vi "Get Process LLB Actions.vi"(8 "error in (no error)":errorcluster {"code" format="Error %.0f"}, 11 "VIDoc Printer In":refnum<class "VIDoc Printer.lvclass">) -> (0 "error out":errorcluster {"code" format="Error %.0f"}, 2 "Process LLB Actions":T1[](array[typedef]), 3 "VIDoc Printer Out":refnum<class "VIDoc Printer.lvclass">)   [LabVIEW 2023, in "VIDoc Printer.lvlib" / "VIDoc Printer.lvclass"]
uses:
  VIDoc Printer.lvclass
  VIDoc Printer.lvclass/VIDoc Printer.ctl
  Controls/Process LLB Enum.ctl
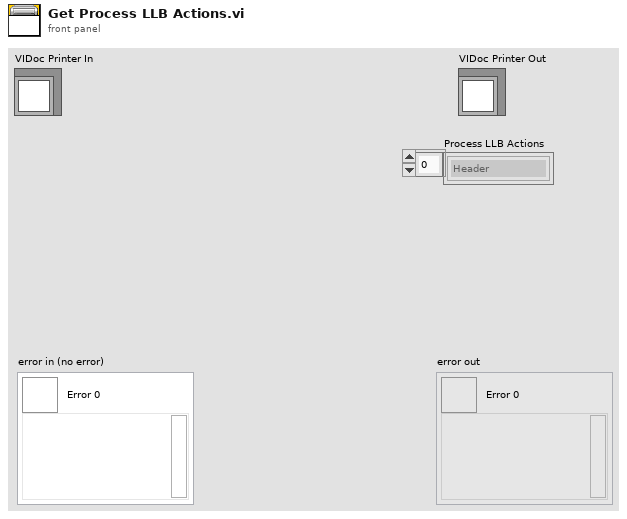
[diagram p1: front panel]
types:
  T1 = typedef "VIDoc Printer.lvlib/VIDoc Printer.lvclass/Process LLB Enum.ctl" = enum16{"Header", "By List", "Methods", "Controls"}
  T2 = typedef "VIDoc Printer.lvlib/Printer Settings.lvclass/Detail Level Enum.ctl" = enum16{"None", "Minimal", "Standard", "Full"}
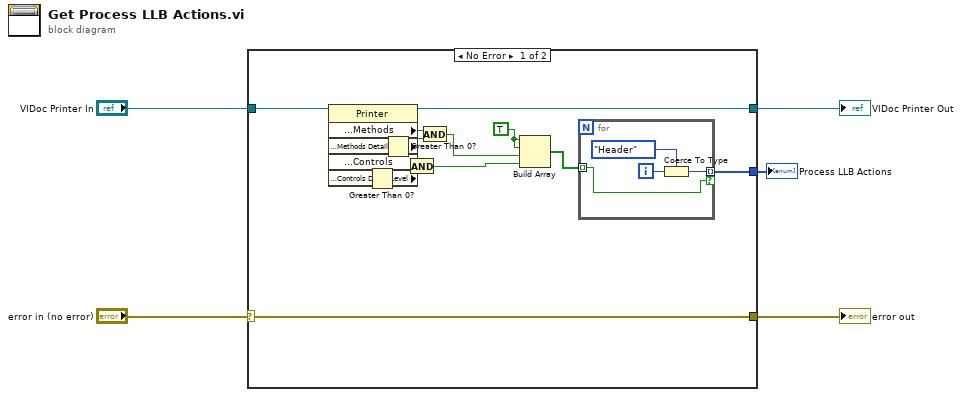
[diagram p0: block diagram]
diagram:
  n1 = case shown="No Error" "error in (no error)" {
    selector: "error in (no error)" -> [w19 w25]
    tunnel: [w19 w25] -> w4
    tunnel: [w16 w24] -> w2
    tunnel: "VIDoc Printer In" -> [w17 w24]
    tunnel: [w14 _] -> w1
    frame No Error {
      w6 = TRUE ("element")
      n2 = property class="Printer"(reference=w17) -> (reference out=w16:refnum<class "VIDoc Printer.lvclass">, "Properties:Settings:LLBs:Methods"=w18:bool, "Properties:Settings:LLBs:Methods Detail Level"=w13:T2, "Properties:Settings:LLBs:Controls"=w10:bool, "Properties:Settings:LLBs:Controls Detail Level"=w8:T2)  [unwired: 1 in, 1 out]
      n3 = Greater Than 0?(x=w8) -> (x > 0?=w9:bool)
      n4 = Greater Than 0?(x=w13) -> (x > 0?=w11:bool)
      n5 = And(x=w10, y=w9) -> (x .and. y?=w7:bool)
      n6 = And(x=w18, y=w11) -> (x .and. y?=w12:bool)
      n7 = Build Array(w6, w6, w12, w7) -> (w15:bool[])
      n8 = for {
        tunnel: w15 -> [w20] mode=indexing
        tunnel: [w21] -> w14 mode=indexing if=w20
        i -> [w22]
        n9 = Coerce To Type(0:w22, 1:Process_LLB_Enum."Header") -> (2:w21:T1)
      }
    }
    frame Error {
    }
  }
  "error out" <- w4
  "VIDoc Printer Out" <- w2
  "Process LLB Actions" <- w1
